vi "BioFeedback15(ModularMeanEnvelope).vi"(7 "Frames Per Second":dbl=30.0, 9 "Start Trial":bool, 11 "End Trial":bool, 12 "Data Directory":path, 13 "File Name":string, 14 "Extension":string="_EMG.txt") -> ()   [LabVIEW 2016]
uses:
  <vilib>/Waveform/WDTOps.llb/WDT Append Waveforms DBL.vi
  <vilib>/Utility/error.llb/DialogType.ctl
  <vilib>/Utility/file.llb/Write Delimited Spreadsheet (string).vi
  <vilib>/Waveform/WDTFileIO.llb/Export Waveforms To Spreadsheet File (1D).vi
  customSubVIs/Control 1.ctl
panel:
  out "Display Buffer":dbl[][](array[numeric])
  out "MVC Buffer Index":dbl=3.0
  out "Display Buffer Index":dbl=3.0
  out "FilteredTrialData One Channel":waveform(dbl)(graph)
  out "Raw Trial Data One  Channel":waveform(dbl)(graph)
  out "DisplayMaxArray":dbl[](array[numeric])
  out "EndProcessTic":u32
  out "StartProcessTic":u32
  out "EndRecordTic":u32
  out "startRecordTic":u32
  out "Start UI":timestamp
  out "UI Elapsed Time":u32
  out "End UI":timestamp
  out "End Process":timestamp
  out "Start Process":timestamp
  out "End Record":timestamp
  out "Start Record":timestamp
  out "Process Elapsed Time":u32
  out "Record Elapsed Time":u32
  out "FilteredTrialData":waveform(dbl)[](graph)
  out "FilteredAndRectified":waveform(dbl)[](graph) caption="Filtered and Rectified"
  out "FilteredDataArray":waveform(dbl)[](array[waveform])
  in  "DisplayChannel":dbl
  out "DisplayTrialData":T1
  out "DisplayValueByChannel":dbl[](array[numeric])
  out "MVCBufferSize":dbl
  in  "MVC Window Size (s)":dbl=0.5
  out "CurrentAvgByChannel":dbl[](array[numeric])
  out "MVC Buffer":dbl[][](array[numeric])
  out "Trial Data Column Headers":string[](array[string])
  in  "TrialDataRowHeaders":string[](array[string])=["Wfm1", "Wfm2", "Wfm3", "Wfm4", "Wfm5", "Wfm6", "Wfm7", "Wfm8"]
  out "GetMaxStartTime":timestamp
  in  "SecondsToAcquireMax":dbl=10.0
  out "MVC Count":dbl=3.0
  out "SignalsMaxArray":dbl[](array[numeric])
  out "RawTrialData":waveform(dbl)[](array[waveform])
  in  "UI Ampl Error Path":path=path "C:/Users/Tinggroup/Desktop/VRMuscleActivationVisualizer/VRBiofeedback_v2/assets/BiofeedbackAmplitudeError.txt"
  out "DisplayActivation":dbl
  out "Get MVC":bool
  in  "resetMax":bool
  in  "startGetMax":bool
  in  "Amplitude Error":dbl
  in  "UI Data Path":path=path "C:/Users/Tinggroup/Desktop/VRMuscleActivationVisualizer/VRBiofeedback_v2/assets/LeftEMGData.txt"
  in  "EMG Input Device\nProduct Type":string="USB-6009"
  out "DisplayBarActivation":dbl(slide) caption="Left" max=1.0 scale=0.0..100.0
  out "NormalizedSignal8":dbl[](graph)
  out "NormalizedSignal7":dbl[](graph)
  out "NormalizedSignal6":dbl[](graph)
  out "NormalizedSignal5":dbl[](graph)
  out "NormalizedSignal4":dbl[](graph)
  out "NormalizedSignal3":dbl[](graph)
  out "NormalizedSignal2":dbl[](graph)
  out "NormalizedSignal1":dbl[](graph)
  out "Raw Trial Data Wfm":waveform(dbl)[](graph)
  in  "UI Percent Path":path=path "C:/Users/Tinggroup/Desktop/VRMuscleActivationVisualizer/VRBiofeedback_v2/assets/BiofeedbackTargetPercentage.txt"
  in  "Target Percentage":dbl=10.0
  out "Trial In Progress":bool
  in  "Lower Cut-Off":dbl=20.0
  in  "Upper Cut-Off":dbl=300.0
  out "raw data":dynamicdata(graph)
  out "DisplayBufferSize":dbl
  out "Samples per frame":dbl
  out "Reset":bool=TRUE
  in  "Display Window Size (s)":dbl=0.02
  in  "Sample rate (Hz)":dbl=2000.0
  in  "End Program":bool
  # "Data To Be Saved (Not including Max Data)"
  # "Performance Metrics"
  # "Saving Trial Data"
  # "Small Window"
  # "Set Target"
  # "Scale Max"
  # "Filter and Process Parameters"
  # "MVC Scaling Variables"
  # "Start and end recording for max?"
  # "Big Window"
  # "Display Parameters"
  # "Changes are made instantly and cause moving average to reset to zero"
  # "Analyze Stability of Displayed Data (Not Functional)"
  # "Auto Analyze Stability begins calculating stability\nAs soon as dot enters the target zone and stops \nonce the dot leaves the target zone (Not Yet Implemented)"
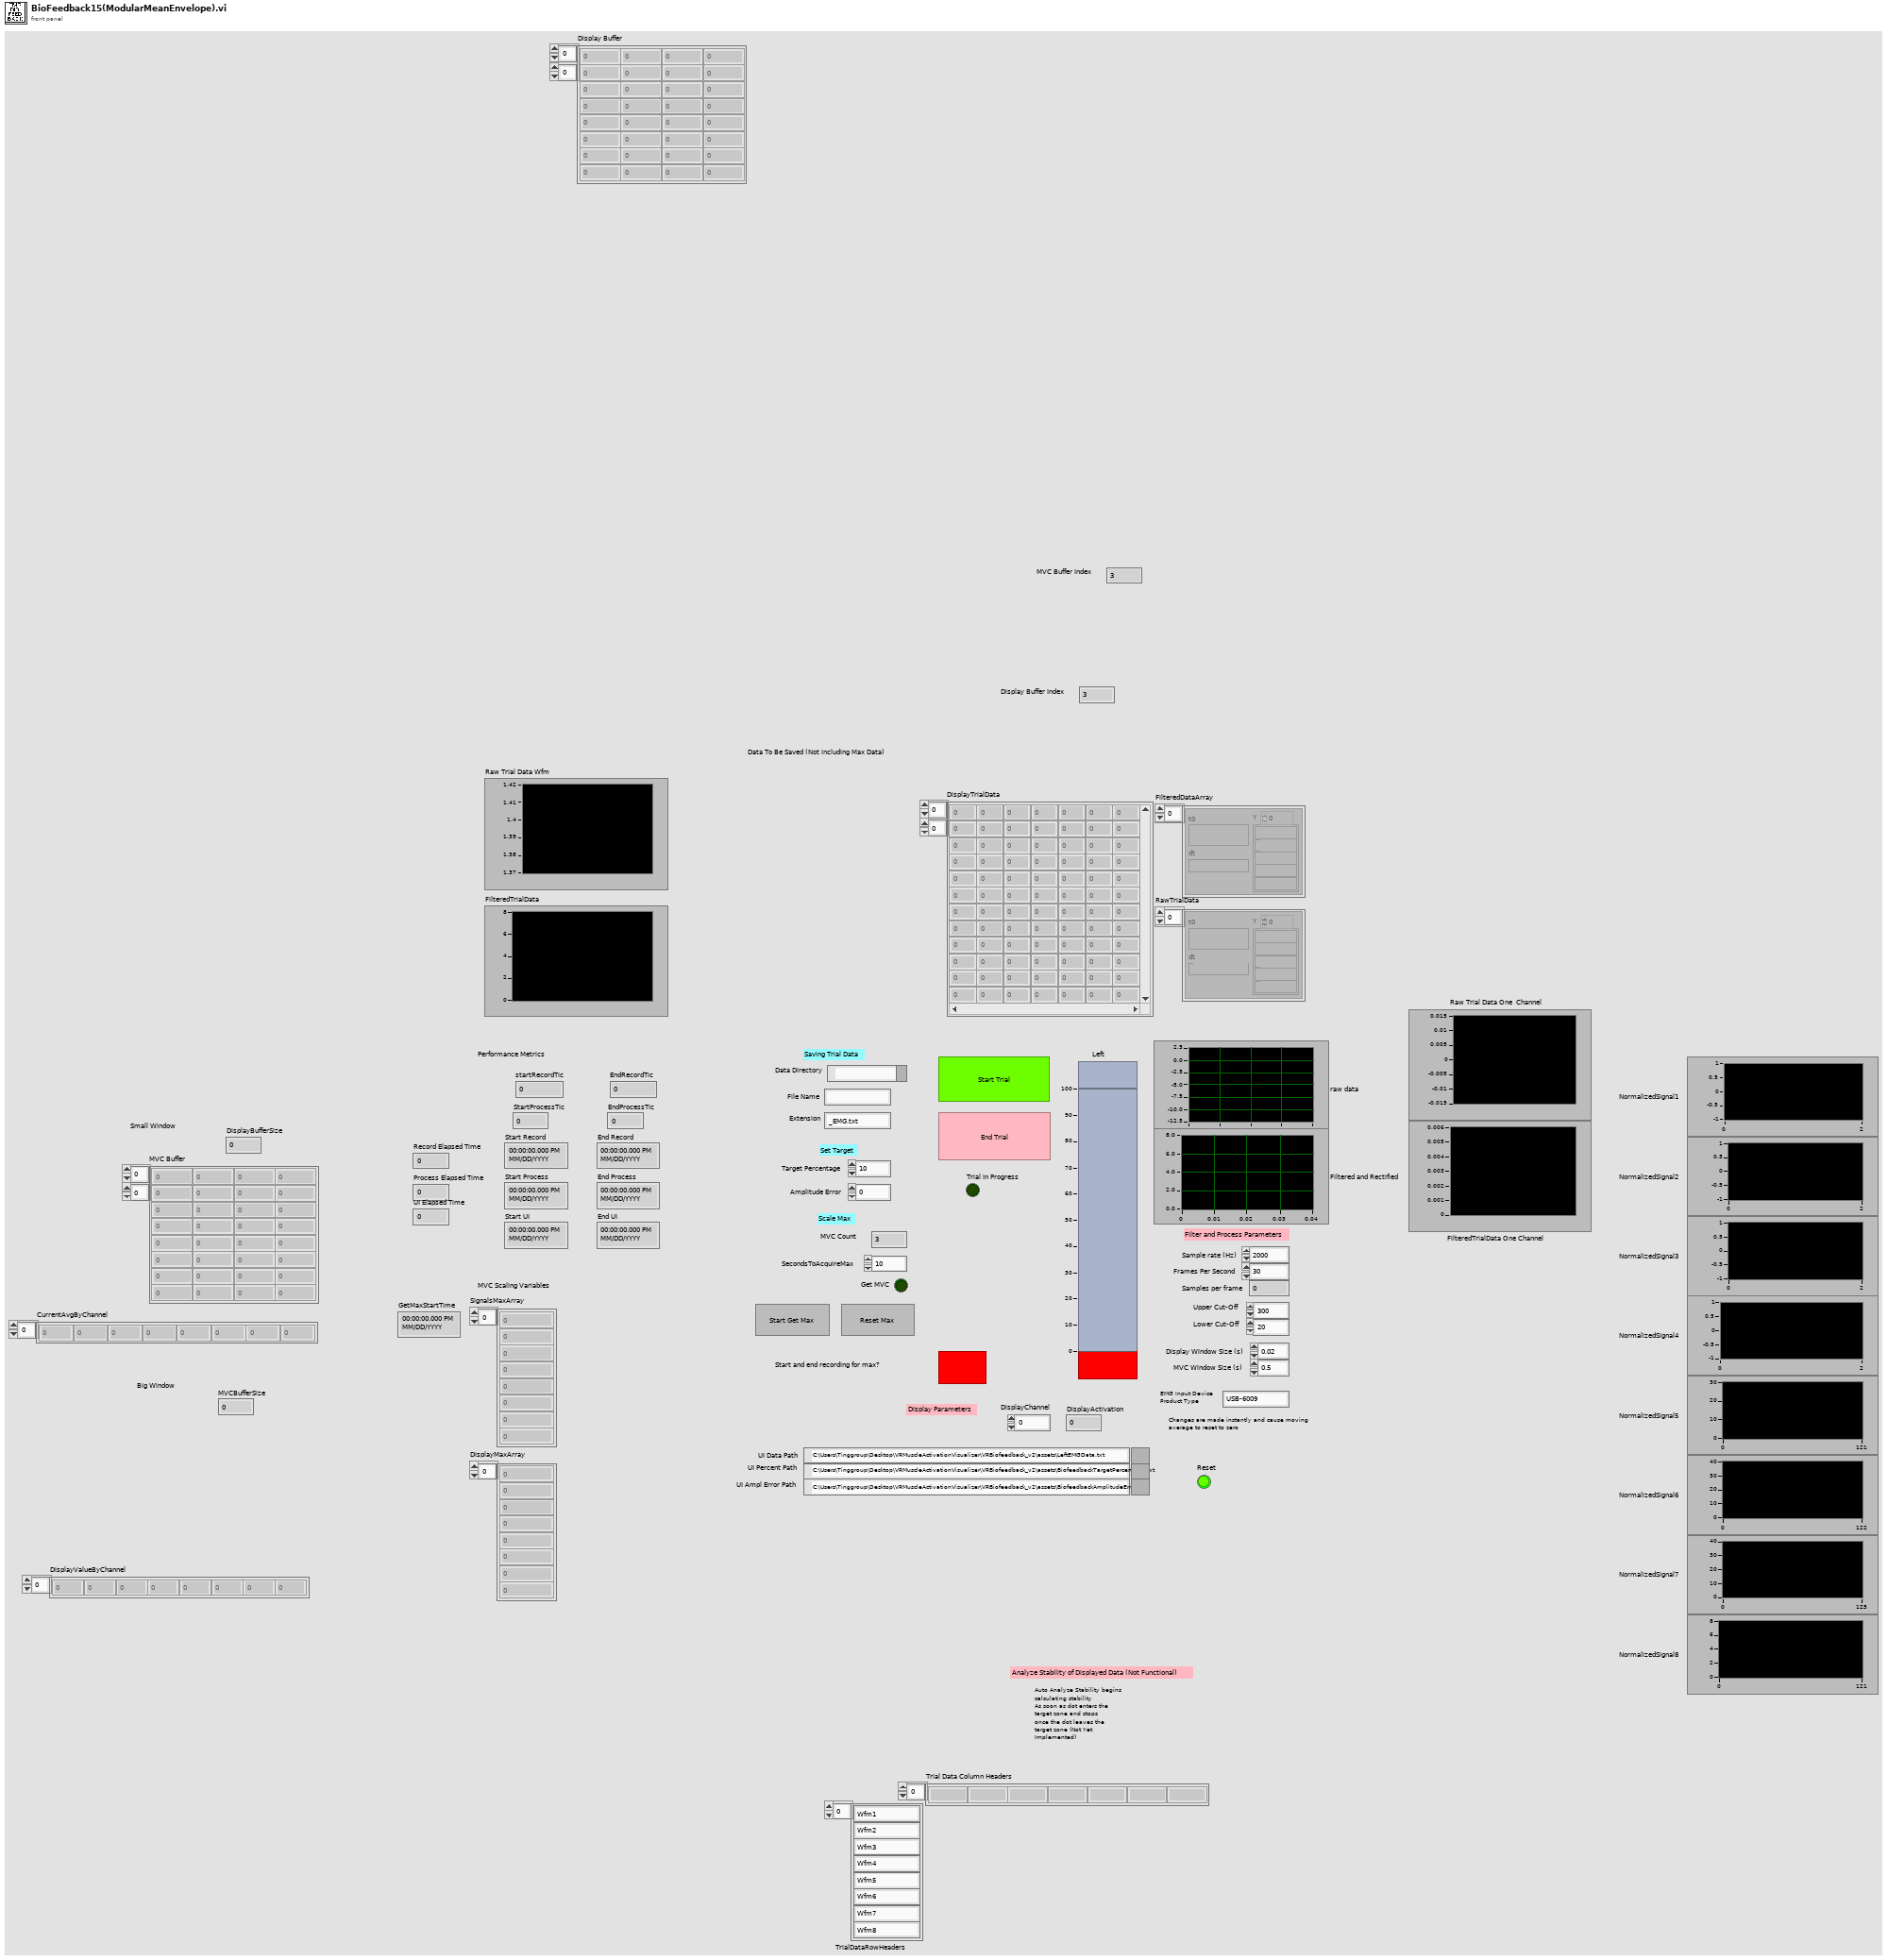
[diagram p1: front panel]
types:
  T1 = typedef "Control 1.ctl" = dbl[][]
  T2 = typedef "DialogType.ctl" = u16
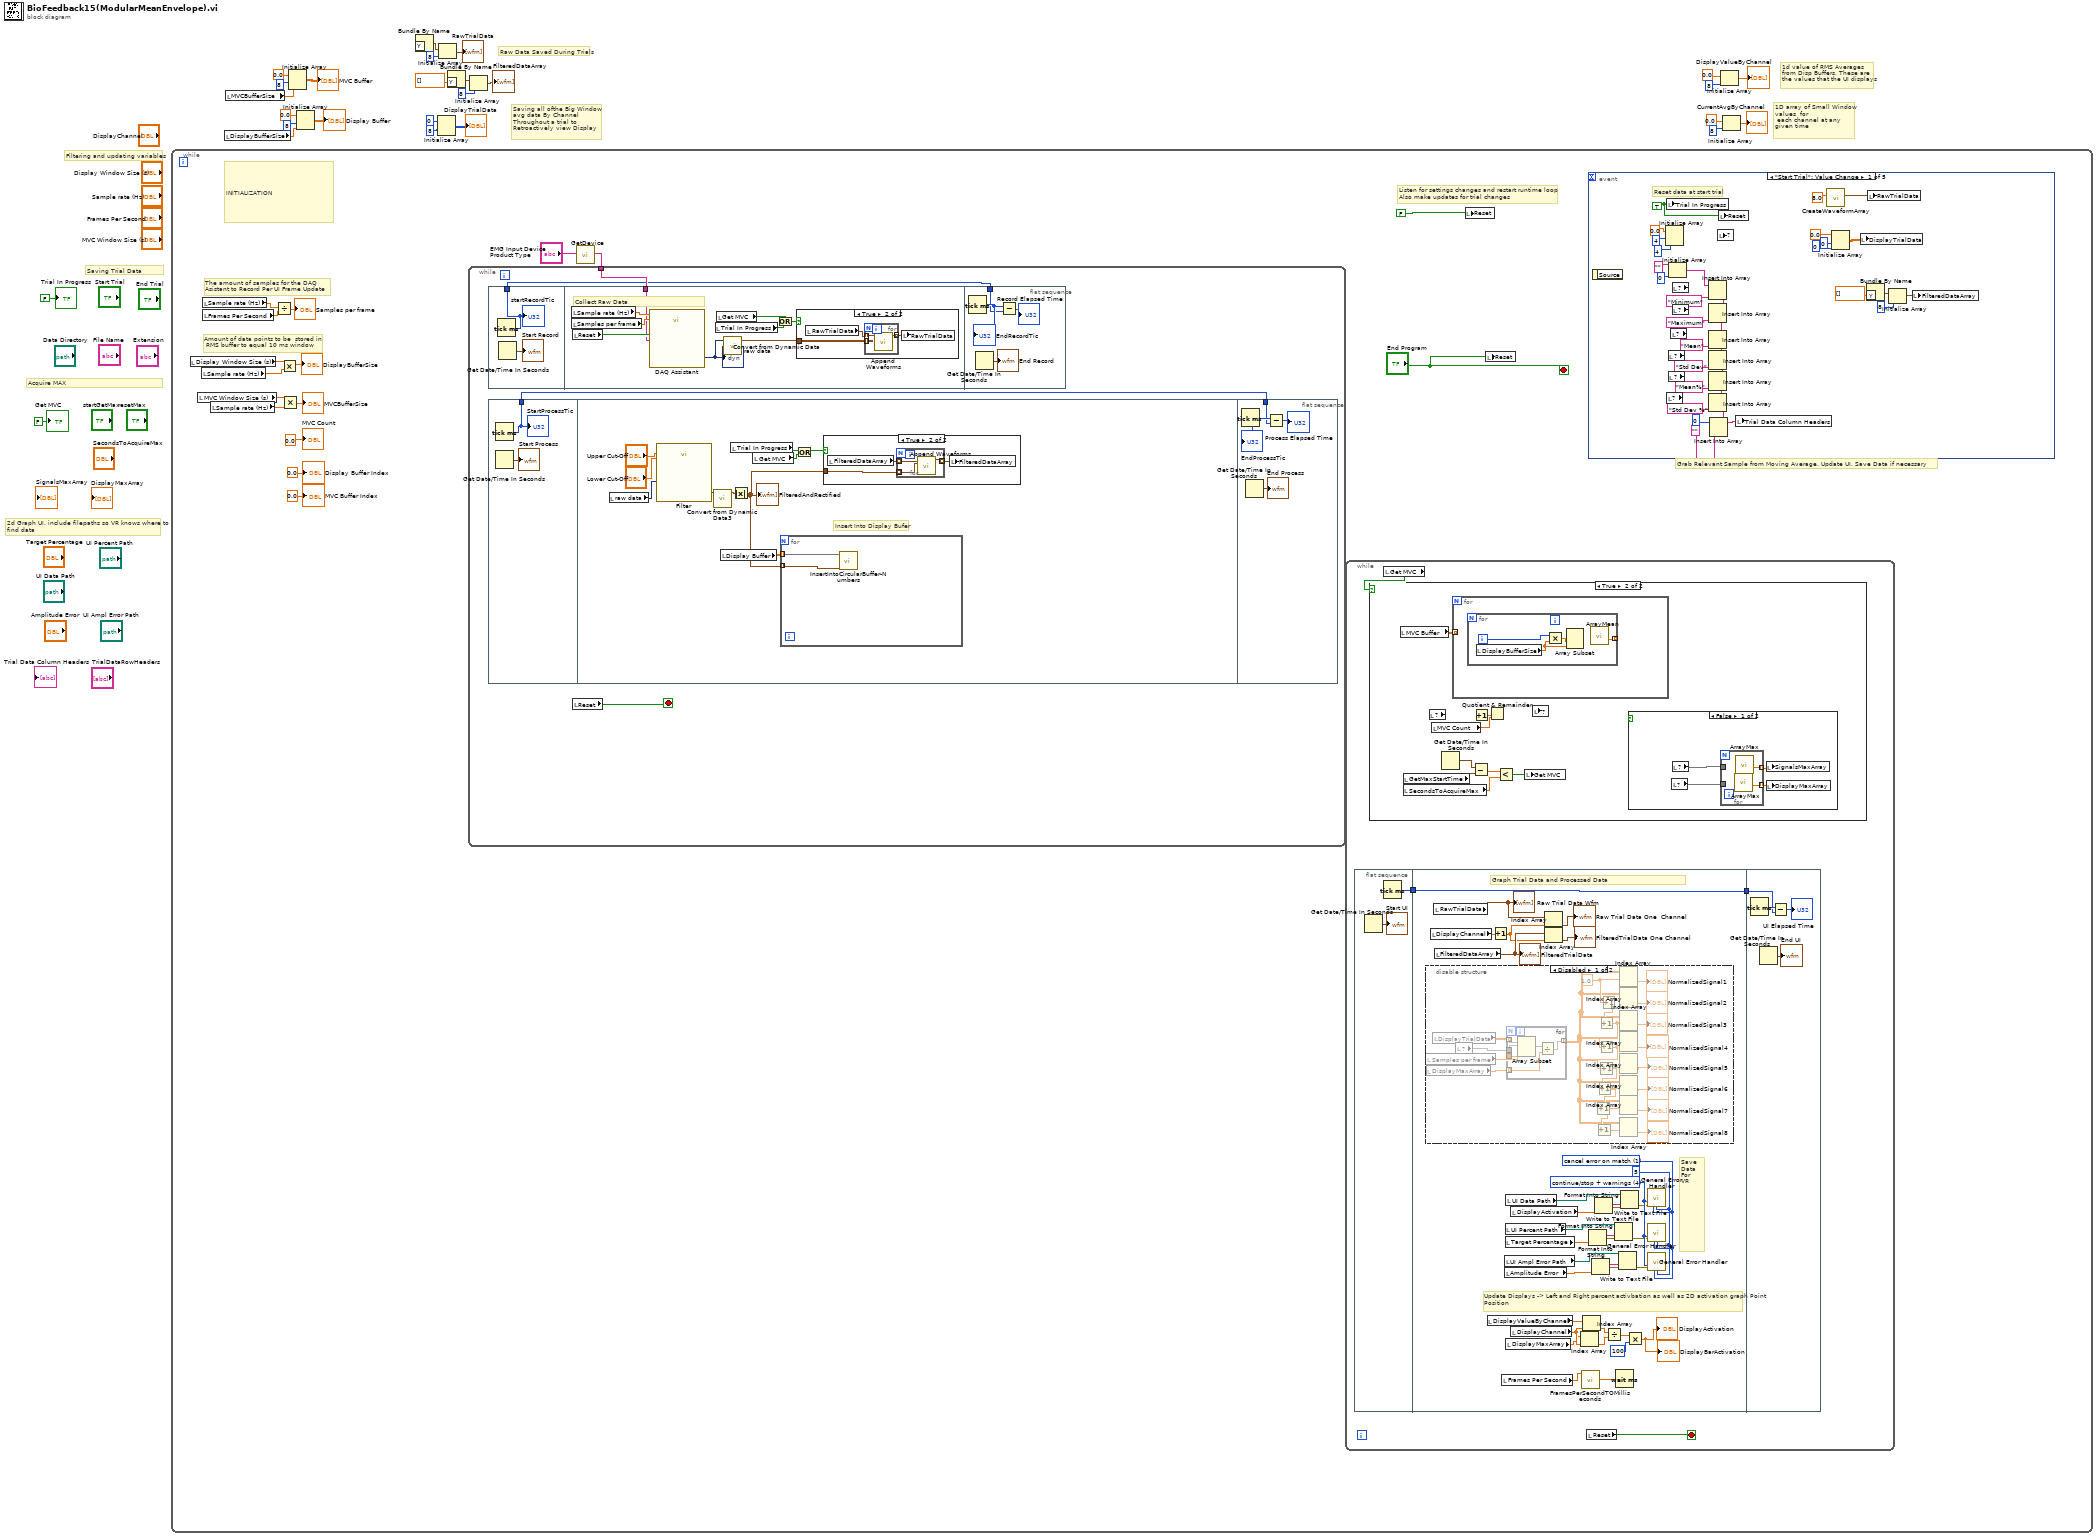
[diagram p0: block diagram]
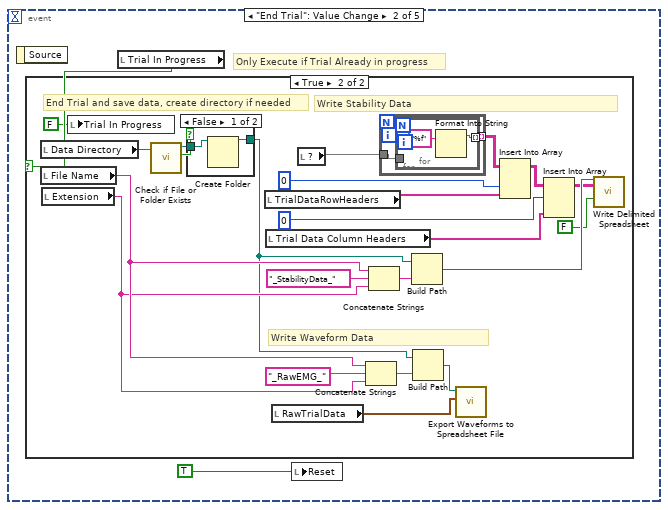
[diagram p5: hidden frame]
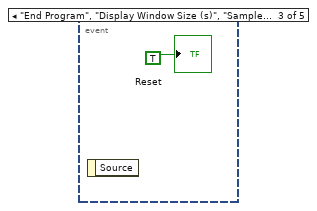
[diagram p8: hidden frame]
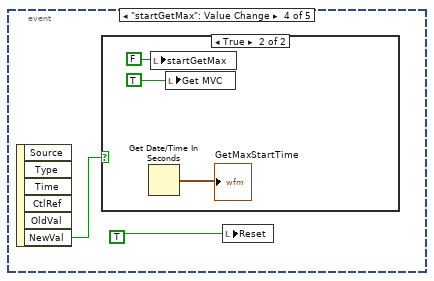
[diagram p9: hidden frame]
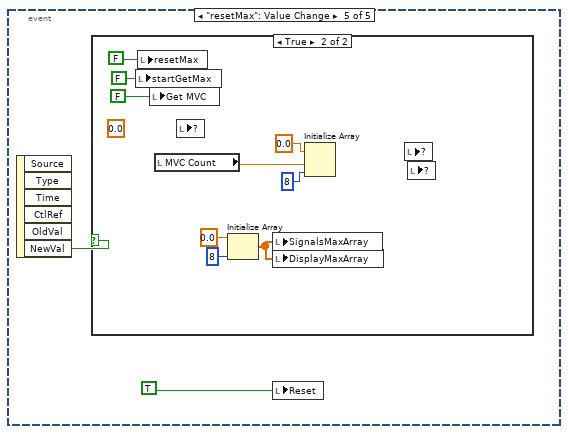
[diagram p11: hidden frame]
diagram:
  # "Saving all ofthe Big Window \navg data By Channel\nThroughout a trial to \nRetroactively view Display"
  # "1d value of RMS Averages\nfrom Disp Buffers. These are\nthe values that the UI displays"
  # "1D array of Small Window\nvalues  for\n each channel at any\ngiven time"
  # "Raw Data Saved During Trials"
  # "Acquire MAX"
  # "Filtering and updating variables"
  # "Saving Trial Data"
  # "2d Graph UI, include filepaths so VR knows where to find data"
  n1 = while {
    stop <- "End Program" stop-if-true
    # "INITIALIZATION"
    # "Grab Relevant Sample from Moving Average, Update UI, Save Data if necessary"
    # "Amount of data points to be  stored in\n RMS buffer to equal 10 ms window"
    # "The amount of samples for the DAQ Asistant to Record Per UI Frame Update"
    # "Listen for settings changes and restart runtime loop\nAlso make updates for trial changes"
    n2 = local read "Display Window Size (s)"() -> (w35:dbl)
    n3 = local read "MVC Window Size (s)"() -> (w31:dbl)
    n4 = local read "Sample rate (Hz)"() -> (w36:dbl)
    n5 = local read "Sample rate (Hz)"() -> (w42:dbl)
    n6 = local read "Frames Per Second"() -> (w41:dbl)
    n7 = local read "Sample rate (Hz)"() -> (w29:dbl)
    n8 = Divide(x=w42, y=w41) -> (x/y=→"Samples per frame":dbl)
    n9 = Multiply(x=w35, y=w36) -> (x*y=→"DisplayBufferSize":dbl)
    n10 = Multiply(x=w31, y=w29) -> (x*y=→"MVCBufferSize":dbl)
    n11 = call "GetDevice.vi"("EMG Input Device\nProduct Type"="EMG Input Device\nProduct Type") -> ("DAQmx Device Name"=w37:tag)  [unwired: 10 in]
    n12 = while {
      tunnel: w37 -> [w217]
      stop <- w216 stop-if-true
      n13 = flat-sequence {
        tunnel: [w243] -> w214
        tunnel: w217 -> [w248]
        tunnel: w214 -> [w259]
        frame #0 {
          n14 = Tick Count (ms)() -> (millisecond timer value=w243:u32)
          "startRecordTic" <- w243
          n15 = Get Date/Time In Seconds() -> (seconds since 1Jan1904=→"Start Record":timestamp)
        }
        frame #1 {
          # "Collect Raw Data"
          n16 = local read "Sample rate (Hz)"() -> (w251:dbl)
          n17 = local read "Samples per frame"() -> (w250:dbl)
          n18 = local read "Reset"() -> (w249:bool)
          n19 = call "DAQ Assistant"("rate"=w251, "number of samples"=w250, "stop (T)"=w249, "device name"=w248) -> ("data"=w245:dynamicdata)  [unwired: 13 in, 2 out]
          "raw data" <- w245
          n20 = local read "Trial In Progress"() -> (w247:bool)
          n21 = local read "Get MVC"() -> (w246:bool)
          n22 = call "Convert from Dynamic Data"("Dynamic Data Type"=w245) -> ("Array of Waveform"=w252:waveform(dbl)[])  [unwired: 3 in]
          n23 = Or(x=w246, y=w247) -> (x .or. y?=w244:bool)
          n24 = case shown="True" w244 {
            tunnel: w252 -> [_ w255]
            frame False {
            }
            frame True {
              n25 = local read "RawTrialData"() -> (w253:waveform(dbl)[])
              n26 = for {
                tunnel: w255 -> [w257] mode=indexing
                tunnel: w253 -> [w258] mode=indexing
                tunnel: [w256] -> w254 mode=indexing
                n27 = call-poly <vilib>:"Append Waveforms.vi"("waveform B"=w257, "waveform A"=w258) -> ("waveform out"=w256:waveform(dbl))  [unwired: 8 in, 1 out]
              }
              n28 = local write "RawTrialData"(w254) -> ()
            }
          }
        }
        frame #2 {
          n29 = Tick Count (ms)() -> (millisecond timer value=w260:u32)
          "EndRecordTic" <- w260
          n30 = Get Date/Time In Seconds() -> (seconds since 1Jan1904=→"End Record":timestamp)
          n31 = Subtract(x=w260, y=w259) -> (x-y=→"Record Elapsed Time":u32)
        }
      }
      n32 = flat-sequence {
        tunnel: [w219] -> w215
        tunnel: w215 -> [w239]
        frame #0 {
          n33 = Get Date/Time In Seconds() -> (seconds since 1Jan1904=→"Start Process":timestamp)
          n34 = Tick Count (ms)() -> (millisecond timer value=w219:u32)
          "StartProcessTic" <- w219
        }
        frame #1 {
          # "Insert Into Display Bufer"
          n35 = local read "raw data"() -> (w223:dynamicdata)
          n36 = call "Filter"("Lower Cut-Off"="Lower Cut-Off", "Upper Cut-Off"="Upper Cut-Off", "Signal"=w223) -> ("Filtered Signal"=w229:dynamicdata)  [unwired: 7 in, 1 out]
          n37 = call "Convert from Dynamic Data3"("Dynamic Data Type"=w229) -> ("Array of Waveform"=w228:waveform(dbl)[])  [unwired: 3 in]
          n38 = local read "Display Buffer"() -> (w221:dbl[][])
          n39 = local read "Trial In Progress"() -> (w225:bool)
          n40 = Absolute Value(x=w228) -> (abs(x)=w220:waveform(dbl)[])
          "FilteredAndRectified" <- w220
          n41 = local read "Get MVC"() -> (w222:bool)
          n42 = for {
            tunnel: w221 -> [w231] mode=indexing
            tunnel: w220 -> [w230] mode=indexing
            n43 = call "InsertIntoCircularBuffer-Numbers.vi"("NewElements"=w230, "Buffer"=w231) -> ()  [unwired: 8 in, 2 out]
          }
          n44 = Or(x=w225, y=w222) -> (x .or. y?=w224:bool)
          n45 = case shown="True" w224 {
            tunnel: w220 -> [_ w233]
            frame False {
            }
            frame True {
              n46 = local read "FilteredDataArray"() -> (w234:waveform(dbl)[])
              n47 = for {
                tunnel: w234 -> [w237] mode=indexing
                tunnel: w233 -> [w236] mode=indexing
                tunnel: [w235] -> w232 mode=indexing
                n48 = call-poly <vilib>:"Append Waveforms.vi"("waveform B"=w236, "waveform A"=w237) -> ("waveform out"=w235:waveform(dbl))  [unwired: 8 in, 1 out]
              }
              n49 = local write "FilteredDataArray"(w232) -> ()
            }
          }
        }
        frame #2 {
          n50 = Tick Count (ms)() -> (millisecond timer value=w240:u32)
          "EndProcessTic" <- w240
          n51 = Get Date/Time In Seconds() -> (seconds since 1Jan1904=→"End Process":timestamp)
          n52 = Subtract(x=w240, y=w239) -> (x-y=→"Process Elapsed Time":u32)
        }
      }
      n53 = local read "Reset"() -> (w216:bool)
    }
    n54 = while {
      stop <- w44 stop-if-true
      n55 = flat-sequence {
        tunnel: [w66] -> w46
        tunnel: [w101] -> w45
        tunnel: w46 -> [w101]
        tunnel: w45 -> [w129]
        frame #0 {
          n56 = Get Date/Time In Seconds() -> (seconds since 1Jan1904=→"Start UI":timestamp)
          n57 = Tick Count (ms)() -> (millisecond timer value=w66:u32)
        }
        frame #1 {
          w96 = T2 4 items=["no dialog", "OK message", "continue or stop message", "OK message + warnings", "continue/stop + warnings"] ("type of dialog (OK msg:1)")
          w97 = 1 items=["no exception", "cancel error on match", "set error on match"] ("[exception action] (none:0)")
          w98 = 5 ("[exception code]")
          # "Graph Trial Data and Processed Data"
          # "Update Displays -> Left and Right percent activbation as well as 2D activation graph Point Position"
          # "Save\nData\nFor\nVR"
          n58 = disable-structure shown="Disabled" {
            frame Disabled {
              w122 = 1.0 ("x")
              n59 = local read "Samples per frame"() -> (w103:dbl)
              n60 = local read "DisplayMaxArray"() -> (w102:dbl[])
              n61 = local read "DisplayTrialData"() -> (w105:T1)
              n62 = local read item#-1() -> (w104)
              n63 = for {
                tunnel: w105 -> [w127] mode=indexing
                tunnel: w102 -> [w123] mode=indexing
                tunnel: [w128] -> w106 mode=indexing
                tunnel: w104 -> [w126]
                tunnel: w103 -> [w125]
                n64 = Array Subset(array=w127, index=w126, length=w125) -> (w124:dbl[])
                n65 = Divide(x=w124, y=w123) -> (x/y=w128:dbl[])
              }
              n66 = Increment(x=w122) -> (x+1=w121:dbl)
              n67 = Increment(x=w121) -> (x+1=w120:dbl)
              n68 = Increment(x=w120) -> (x+1=w119:dbl)
              n69 = Increment(x=w119) -> (x+1=w118:dbl)
              n70 = Increment(x=w118) -> (x+1=w117:dbl)
              n71 = Increment(x=w117) -> (x+1=w116:dbl)
              n72 = Increment(x=w116) -> (x+1=w115:dbl)
              n73 = Index Array(array=w106, index (row)=w122) -> (element=→"NormalizedSignal1":dbl[])  [unwired: 1 in]
              n74 = Index Array(array=w106, index (row)=w121) -> (element=→"NormalizedSignal2":dbl[])  [unwired: 1 in]
              n75 = Index Array(array=w106, index (row)=w120) -> (element=→"NormalizedSignal3":dbl[])  [unwired: 1 in]
              n76 = Index Array(array=w106, index (row)=w119) -> (element=→"NormalizedSignal4":dbl[])  [unwired: 1 in]
              n77 = Index Array(array=w106, index (row)=w118) -> (element=→"NormalizedSignal5":dbl[])  [unwired: 1 in]
              n78 = Index Array(array=w106, index (row)=w117) -> (element=→"NormalizedSignal6":dbl[])  [unwired: 1 in]
              n79 = Index Array(array=w106, index (row)=w116) -> (element=→"NormalizedSignal7":dbl[])  [unwired: 1 in]
              n80 = Index Array(array=w106, index (row)=w115) -> (element=→"NormalizedSignal8":dbl[])  [unwired: 1 in]
            }
            frame Enabled {
            }
          }
          n81 = local read "DisplayChannel"() -> (w72:dbl)
          n82 = local read "RawTrialData"() -> (w71:waveform(dbl)[])
          "Raw Trial Data Wfm" <- w71
          n83 = local read "FilteredDataArray"() -> (w70:waveform(dbl)[])
          "FilteredTrialData" <- w70
          n84 = local read "DisplayValueByChannel"() -> (w100:dbl[])
          n85 = Increment(x=w72) -> (x+1=w69:dbl)
          n86 = local read "Frames Per Second"() -> (w78:dbl)
          n87 = local read "UI Ampl Error Path"() -> (w95:path)
          n88 = local read "Amplitude Error"() -> (w94:dbl)
          n89 = local read "UI Percent Path"() -> (w87:path)
          n90 = local read "Target Percentage"() -> (w88:dbl)
          n91 = local read "UI Data Path"() -> (w81:path)
          n92 = local read "DisplayMaxArray"() -> (w73:dbl[])
          n93 = local read "DisplayActivation"() -> (w83:dbl)
          n94 = local read "DisplayChannel"() -> (w74:dbl)
          n95 = Index Array(array=w71, index=w69) -> (element=→"Raw Trial Data One  Channel":waveform(dbl))
          n96 = Index Array(array=w70, index=w69) -> (element=→"FilteredTrialData One Channel":waveform(dbl))
          n97 = Index Array(array=w73, index=w74) -> (element=w75:dbl)
          n98 = call "FramesPerSecondTOMilliseconds.vi"("Thermometer\nFps"=w78) -> ("x*y"=w99:dbl)  [unwired: 10 in]
          n99 = Index Array(array=w100, index=w74) -> (element=w77:dbl)
          n100 = Format Into String(w88) -> (resulting string=w86:string, error out=w85:errorcluster)  [unwired: 3 in]
          n101 = Format Into String(w94) -> (resulting string=w93:string, error out=w92:errorcluster)  [unwired: 3 in]
          n102 = Format Into String(w83) -> (resulting string=w82:string, error out=w80:errorcluster)  [unwired: 3 in]
          n103 = Divide(x=w77, y=w75) -> (x/y=w90:dbl)
          n104 = Write to Text File(file (use dialog)=w87, text=w86, error in=w85) -> (error out=w84:errorcluster)  [unwired: 1 in, 2 out]
          n105 = Wait (ms)(milliseconds to wait=w99) -> ()  [unwired: 1 out]
          n106 = Write to Text File(file (use dialog)=w95, text=w93, error in=w92) -> (error out=w91:errorcluster)  [unwired: 1 in, 2 out]
          n107 = Write to Text File(file (use dialog)=w81, text=w82, error in=w80) -> (error out=w79:errorcluster)  [unwired: 1 in, 2 out]
          n108 = Multiply(x=w90, y=100) -> (x*y=→"DisplayBarActivation" →"DisplayActivation":dbl)
          n109 = call <vilib>:"General Error Handler.vi"("type of dialog (OK msg:1)"=w96, "error in (no error)"=w79, "[exception action] (none:0)"=w97, "[exception code]"=w98) -> ()  [unwired: 7 in, 5 out]
          n110 = call <vilib>:"General Error Handler.vi"("type of dialog (OK msg:1)"=w96, "error in (no error)"=w84, "[exception action] (none:0)"=w97, "[exception code]"=w98) -> ()  [unwired: 7 in, 5 out]
          n111 = call <vilib>:"General Error Handler.vi"("type of dialog (OK msg:1)"=w96, "error in (no error)"=w91, "[exception action] (none:0)"=w97, "[exception code]"=w98) -> ()  [unwired: 7 in, 5 out]
        }
        frame #2 {
          n112 = Tick Count (ms)() -> (millisecond timer value=w130:u32)
          n113 = Get Date/Time In Seconds() -> (seconds since 1Jan1904=→"End UI":timestamp)
          n114 = Subtract(x=w130, y=w129) -> (x-y=→"UI Elapsed Time":u32)
        }
      }
      n115 = local read "Get MVC"() -> (w43:bool)
      n116 = case shown="True" w43 {
        frame False {
        }
        frame True {
          n117 = local read "MVC Buffer"() -> (w47:dbl[][])
          n118 = local read "GetMaxStartTime"() -> (w54:timestamp)
          n119 = local read "SecondsToAcquireMax"() -> (w51:dbl)
          n120 = local read item#-1() -> ()  [unwired: 1 out]
          n121 = local read "MVC Count"() -> (w48:dbl)
          n122 = Get Date/Time In Seconds() -> (seconds since 1Jan1904=w53:timestamp)
          n123 = for {
            tunnel: w47 -> [_] mode=indexing
            n124 = for {
              tunnel: [w55] -> _ mode=indexing
              i -> [w56]
              n125 = local read "DisplayBufferSize"() -> (w57:dbl)
              n126 = Multiply(x=w56, y=w57) -> (x*y=w58:dbl)
              n127 = Array Subset(index=w58, length=w57) -> ()  [unwired: 1 in, 1 out]
              n128 = call "ArrayMean.vi"() -> ("Mean"=w55:dbl)  [unwired: 11 in]
            }
          }
          n129 = Subtract(x=w53, y=w54) -> (x-y=w52:dbl)
          n130 = Increment() -> (x+1=w49:dbl)  [unwired: 1 in]
          n131 = Quotient & Remainder(x=w49, y=w48) -> ()  [unwired: 2 out]
          n132 = Less?(x=w52, y=w51) -> (x < y?=w50:bool)
          n133 = local write "Get MVC"(w50) -> ()
          n134 = local read item#-1() -> ()  [unwired: 1 in]
          n135 = case shown="False" {
            selector: _ -> [_ _]
            frame False {
              n136 = local read item#-1() -> (w60)
              n137 = local read item#-1() -> (w62)
              n138 = for {
                tunnel: w62 -> [_]
                tunnel: [w64] -> w61 mode=indexing
                tunnel: w60 -> [_]
                tunnel: [w63] -> w59 mode=indexing
                n139 = call "ArrayMax.vi"() -> ("max"=w63:dbl)  [unwired: 11 in]
                n140 = call "ArrayMax.vi"() -> ("max"=w64:dbl)  [unwired: 11 in]
              }
              n141 = local write "SignalsMaxArray"(w61) -> ()
              n142 = local write "DisplayMaxArray"(w59) -> ()
            }
            frame True {
            }
          }
        }
      }
      n143 = local read "Reset"() -> (w44:bool)
    }
    n144 = local write "Reset"(FALSE) -> ()
    n145 = local write "Reset"("End Program") -> ()
    n146 = event shown="[0] \"Start Trial\": Value Change" {
      selector: _ -> [_ _ _ _ _]
      dyn-events: _ -> [_ _ _ _ _]
      timeout: _ -> [_ _ _ _ _]
      event "Start Trial": Value Change {
        w164 = TRUE ("Trial In Progress")
        # "Reset data at start trial"
        n147 = event-data() -> ()  [unwired: 1 in, 1 out]
        n148 = Initialize Array(0.0 ("element"), 4 ("dimension size"), 4 ("dimension size")) -> ()  [unwired: 1 out]
        n149 = local write "Trial In Progress"(w164) -> ()
        n150 = local read item#-1() -> ()  [unwired: 1 out]
        n151 = local read item#-1() -> ()  [unwired: 1 out]
        n152 = local read item#-1() -> ()  [unwired: 1 out]
        n153 = Initialize Array("", 0 ("dimension size")) -> (w155:string[])
        n154 = local read item#-1() -> ()  [unwired: 1 out]
        n155 = local read item#-1() -> ()  [unwired: 1 out]
        n156 = local read item#-1() -> ()  [unwired: 1 out]
        n157 = Insert Into Array(array=w155, new element="Minimum" ("new element/subarray")) -> (w153:string[])  [unwired: 1 in]
        n158 = Insert Into Array(array=w153, new element="Maximum" ("new element/subarray")) -> (w151:string[])  [unwired: 1 in]
        n159 = Insert Into Array(array=w151, new element="Mean" ("new element/subarray")) -> (w149:string[])  [unwired: 1 in]
        n160 = Insert Into Array(array=w149, new element="Std Dev" ("new element/subarray")) -> (w147:string[])  [unwired: 1 in]
        n161 = Insert Into Array(array=w147, new element="Mean%" ("new element/subarray")) -> (w145:string[])  [unwired: 1 in]
        n162 = Insert Into Array(array=w145, new element="Std Dev %" ("new element/subarray")) -> (w142:string[])  [unwired: 1 in]
        n163 = Insert Into Array(array=w142, index=0, new element="" ("new element/subarray")) -> (w143:string[])
        n164 = local read item#-1() -> ()  [unwired: 1 in]
        n165 = local write "Reset"(w164) -> ()
        n166 = local write "Trial Data Column Headers"(w143) -> ()
        n167 = call "CreateWaveformArray.vi"("bufferSize"=8.0) -> ("initialized array"=w163:waveform(dbl)[])  [unwired: 5 in, 1 out]
        n168 = Initialize Array(0.0 ("element"), 0 ("dimension size"), 0 ("dimension size")) -> (w137:dbl[][])
        n169 = local write "DisplayTrialData"(w137) -> ()
        n170 = Bundle By Name("Y"=dbl[] []) -> (w136:waveform(dbl))  [unwired: 1 in]
        n171 = local write "RawTrialData"(w163) -> ()
        n172 = Initialize Array(w136, 8 ("dimension size")) -> (w133:waveform(dbl)[])
        n173 = local write "FilteredDataArray"(w133) -> ()
      }
      event "End Trial": Value Change {
        # "Only Execute if Trial Already in progress"
        n174 = event-data() -> ()  [unwired: 1 in, 1 out]
        n175 = local read "Trial In Progress"() -> (w166:bool)
        n176 = case shown="True" w166 {
          frame False {
          }
          frame True {
            # "Write Waveform Data"
            # "Write Stability Data"
            # "End Trial and save data, create directory if needed"
            n177 = local read "Data Directory"() -> (w186:path)
            n178 = local read "File Name"() -> (w172:string)
            n179 = local read "Extension"() -> (w171:string)
            n180 = local write "Trial In Progress"(FALSE ("Trial In Progress")) -> ()
            n181 = call <vilib>:"Check if File or Folder Exists.vi"("path"=w186) -> ("file or folder exists?"=w188:bool, "dup path"=w187:path)  [unwired: 8 in, 1 out]
            n182 = case shown="False" w188 {
              tunnel: [w194 w196] -> w170
              tunnel: w187 -> [w195 w196]
              frame False {
                n183 = Create Folder(path (use dialog)=w195) -> (created path=w194:path)  [unwired: 2 in, 2 out]
              }
              frame True {
              }
            }
            n184 = local read "TrialDataRowHeaders"() -> (w181:string[])
            n185 = local read "Trial Data Column Headers"() -> (w182:string[])
            n186 = local read "RawTrialData"() -> (w168:waveform(dbl)[])
            n187 = local read item#-1() -> (w178)
            n188 = Concatenate Strings(w172, "_RawEMG_" ("string"), w171) -> (w169:string)
            n189 = Concatenate Strings(w172, "_StabilityData_" ("string"), w171) -> (w174:string)
            n190 = for {
              tunnel: w178 -> [w191]
              tunnel: [w190] -> w176 mode=indexing
              n191 = for {
                tunnel: w191 -> [_]
                tunnel: [w192] -> w190 mode=indexing
                n192 = Format Into String(format string="%f") -> (resulting string=w192:string)  [unwired: 3 in, 1 out]
              }
            }
            n193 = Build Path(base path=w170, name or relative path=w174) -> (appended path=w184:path)
            n194 = Build Path(base path=w170, name or relative path=w169) -> (appended path=w167:path)
            n195 = call-poly <vilib>:"Export Waveforms to Spreadsheet File.vi"("waveforms"=w168, "file path (dialog if empty)"=w167) -> ()  [unwired: 8 in, 2 out]
            n196 = Insert Into Array(array=w176, index (col)=0 ("index (row)"), new element=w181) -> (w185:string[][])  [unwired: 1 in]
            n197 = Insert Into Array(array=w185, index (row)=0 ("index (col)"), new element=w182) -> (w177:string[][])  [unwired: 1 in]
            n198 = call-poly <vilib>:"Write Delimited Spreadsheet.vi"("file path (dialog if empty)"=w184, "2D data"=w177, "append to file? (new file:F)"=FALSE) -> ()  [unwired: 11 in, 2 out]
          }
        }
        n199 = local write "Reset"(TRUE ("Reset Data Acquisition\nAnd UI Updating")) -> ()
      }
      event "End Program", "Display Window Size (s)", "Sample rate (Hz)", "Frames Per Second": Value Change {
        n200 = event-data() -> ()  [unwired: 1 in, 1 out]
        "Reset" <- TRUE
      }
      event "startGetMax": Value Change {
        n201 = event-data() -> ("NewVal"=w199:bool)  [unwired: 1 in, 5 out]
        n202 = case shown="True" w199 {
          frame False {
          }
          frame True {
            n203 = Get Date/Time In Seconds() -> (seconds since 1Jan1904=→"GetMaxStartTime":timestamp)
            n204 = local write "startGetMax"(FALSE) -> ()
            n205 = local write "Get MVC"(TRUE ("Acquiring Max")) -> ()
          }
        }
        n206 = local write "Reset"(TRUE ("Reset Data Acquisition\nAnd UI Updating")) -> ()
      }
      event "resetMax": Value Change {
        n207 = event-data() -> ("NewVal"=w204:bool)  [unwired: 1 in, 5 out]
        n208 = case shown="True" w204 {
          frame False {
          }
          frame True {
            (unwired) 0.0 ("CurrentMaxIndex")
            n209 = local write "startGetMax"(FALSE ("startGetMax")) -> ()
            n210 = local write "resetMax"(FALSE ("endGetMax")) -> ()
            n211 = local write "Get MVC"(FALSE ("Acquiring Max")) -> ()
            n212 = local read "MVC Count"() -> (w209:dbl)
            n213 = local read item#-1() -> ()  [unwired: 1 in]
            n214 = Initialize Array(0.0 ("element"), 8 ("dimension size")) -> (w205:dbl[])
            n215 = local write "SignalsMaxArray"(w205) -> ()
            n216 = local write "DisplayMaxArray"(w205) -> ()
            n217 = Initialize Array(0.0 ("element"), w209, 8 ("dimension size")) -> ()  [unwired: 1 out]
            n218 = local read item#-1() -> ()  [unwired: 1 in]
            n219 = local read item#-1() -> ()  [unwired: 1 in]
          }
        }
        n220 = local write "Reset"(TRUE ("Reset Data Acquisition\nAnd UI Updating")) -> ()
      }
    }
    "MVC Count" <- 0.0 ("MVC Count")
    "Display Buffer Index" <- 0.0 ("Display Buffer Index")
    "MVC Buffer Index" <- 0.0 ("MVC Buffer Index")
  }
  n221 = local read "DisplayBufferSize"() -> (w1:dbl)
  n222 = local read "MVCBufferSize"() -> (w19:dbl)
  n223 = Initialize Array(0.0 ("element"), 8 ("dimension size"), w19) -> (→"MVC Buffer":dbl[][])
  n224 = Initialize Array(0.0 ("element"), 8 ("dimension size"), w1) -> (→"Display Buffer":dbl[][])
  n225 = Bundle By Name() -> (w14:waveform(dbl))  [unwired: 2 in]
  n226 = Initialize Array(0, 8 ("dimension size")) -> (→"DisplayTrialData":i32[][])  [unwired: 1 in]
  n227 = Initialize Array(w14, 8 ("dimension size")) -> (→"RawTrialData":waveform(dbl)[])
  n228 = Bundle By Name("Y"=dbl[] []) -> (w6:waveform(dbl))  [unwired: 1 in]
  n229 = Initialize Array(w6, 8 ("dimension size")) -> (→"FilteredDataArray":waveform(dbl)[])
  n230 = Initialize Array(0.0 ("element"), 8 ("dimension size")) -> (→"DisplayValueByChannel":dbl[])
  n231 = Initialize Array(0.0 ("element"), 8 ("dimension size")) -> (→"CurrentAvgByChannel":dbl[])
  "Trial In Progress" <- FALSE ("Trial In Progress")
  "Get MVC" <- FALSE ("Acquiring Max")
